vi "Scan Setup.vi"(8 "error in (no error)":errorcluster, 11 "Wavelength PEM and Digikröm in":refnum<class "Wavelength PEM and Digikröm.lvclass">) -> (0 "error out":errorcluster, 3 "Wavelength PEM and Digikröm out":refnum<class "Wavelength PEM and Digikröm.lvclass">)   [LabVIEW 2017, in "Wavelength PEM and Digikröm.lvclass"]
doc: "Configure the Instrument based on the class member fields. This step comes after the user has closed the \"Scan Setup\" window and before the actual scan -- so instruments are configured with the user's specified settings."
uses:
  Scanner/Scanner.lvclass
  Instruments/Utility Classes/Scannable/Scannable.lvclass
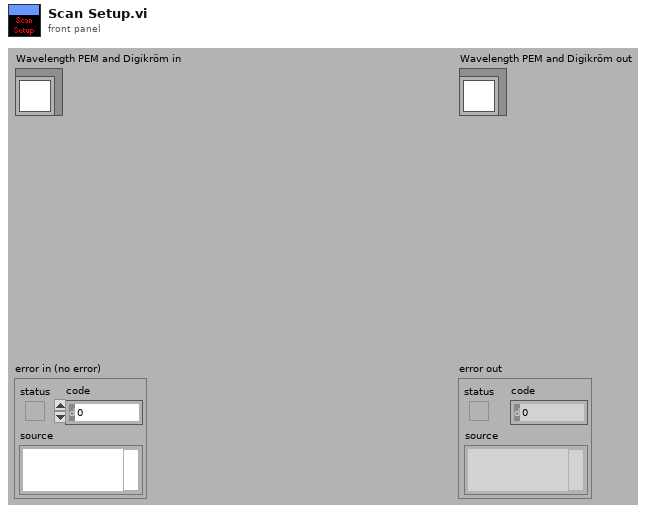
[diagram p1: front panel]
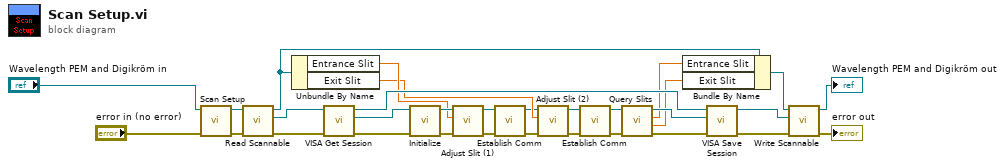
[diagram p0: block diagram]
diagram:
  n1 = call-parent "Scan Setup.vi"("error in (no error)"="error in (no error)", "Scanner in"="Wavelength PEM and Digikröm in") -> ("error out"=w26:errorcluster, "Scanner out"=w29:refnum<class "Wavelength PEM and Digikröm.lvclass">)  [unwired: 8 out]
  n2 = call-dynamic "Read Scannable.vi"("error in (no error)"=w26, "Scanner.lvclass in"=w29) -> ("error out"=w31:errorcluster, "Scannable.lvclass"=w30:refnum<class "Scannable.lvclass">, "Scanner.lvclass out"=w10:refnum<class "Wavelength PEM and Digikröm.lvclass">)  [unwired: 7 out]
  n3 = Unbundle By Name(w10) -> ("Entrance Slit"=w14:dbl[unit], "Exit Slit"=w11:dbl[unit])
  n4 = call-dynamic "VISA Get Session.vi"("error in (no error)"=w31, "Instrument.lvclass in"=w30) -> ("error out"=w25:errorcluster, "VISA Resource Name"=w27:refnum<visa-resource-name>, "Instrument.lvclass out"=w28:refnum<class "Scannable.lvclass">)  [unwired: 7 out]
  n5 = call "Initialize.vi"("error in (no error)"=w25, "VISA resource name"=w27) -> ("error out"=w13:errorcluster, "VISA resource name out"=w16:refnum<visa-resource-name>)  [unwired: 8 out]
  n6 = call "Adjust Slit (1).vi"("error in (no error)"=w13, "SLIT WIDTH"=w14, "VISA resource name"=w16) -> ("error out"=w21:errorcluster, "VISA resource name out"=w22:refnum<visa-resource-name>)  [unwired: 7 out]
  n7 = call "Establish Comm.vi"("error in (no error)"=w21, "VISA resource name"=w22) -> ("error out"=w6:errorcluster, "VISA resource name out"=w7:refnum<visa-resource-name>)  [unwired: 8 in]
  n8 = call "Adjust Slit (2).vi"("error in (no error)"=w6, "SLIT WIDTH"=w11, "VISA resource name"=w7) -> ("error out"=w17:errorcluster, "VISA resource name out"=w18:refnum<visa-resource-name>)  [unwired: 7 out]
  n9 = call "Establish Comm.vi"("error in (no error)"=w17, "VISA resource name"=w18) -> ("error out"=w20:errorcluster, "VISA resource name out"=w19:refnum<visa-resource-name>)  [unwired: 8 in]
  n10 = call "Query Slits.vi"("error in (no error)"=w20, "VISA resource name"=w19) -> ("error out"=w12:errorcluster, "CURRENT S2 WIDTH"=w9:dbl[unit], "CURRENT S1 WIDTH"=w5:dbl[unit], "VISA resource name out"=w15:refnum<visa-resource-name>)  [unwired: 6 out]
  n11 = Bundle By Name(cluster=w10, "Entrance Slit"=w5, "Exit Slit"=w9) -> (w8:refnum<class "Wavelength PEM and Digikröm.lvclass">)
  n12 = call-dynamic "VISA Save Session.vi"("error in (no error)"=w12, "VISA Resource Name"=w15, "Instrument.lvclass in"=w28) -> ("error out"=w24:errorcluster, "Instrument.lvclass out"=w23:refnum<class "Scannable.lvclass">)  [unwired: 7 out]
  n13 = call-dynamic "Write Scannable.vi"("error in (no error)"=w24, "Scannable.lvclass"=w23, "Scanner.lvclass in"=w8) -> ("error out"=→"error out":errorcluster, "Scanner.lvclass out"=→"Wavelength PEM and Digikröm out":refnum<class "Wavelength PEM and Digikröm.lvclass">)  [unwired: 7 out]
